vi "Read from TCP.vi"(8 "error in":errorcluster, 11 "lia host in":refnum<class "LIA Host Interface RT.lvclass">) -> (0 "error out":errorcluster, 3 "lia host out":refnum<class "LIA Host Interface RT.lvclass">)   [LabVIEW 2018, in "LIA Host Interface RT.lvclass"]
uses:
  LIA Host Interface RT.lvclass
  Properties/TcpConnection_GET.vi
  Properties/IncomingQueue_GET.vi
  Properties/LockInQueues_GET.vi
  shared/Lock-In Amplifier Example Shared.lvlib
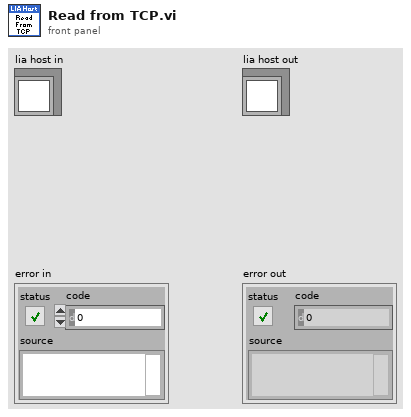
[diagram p1: front panel]
types:
  T1 = enum16{"Standard", "Buffered", "CRLF", "Immediate"}
  T2 = typedef "Lock-In Amplifier Example Shared.lvlib/message.ctl" = cluster{"command":u32, "payload":string}
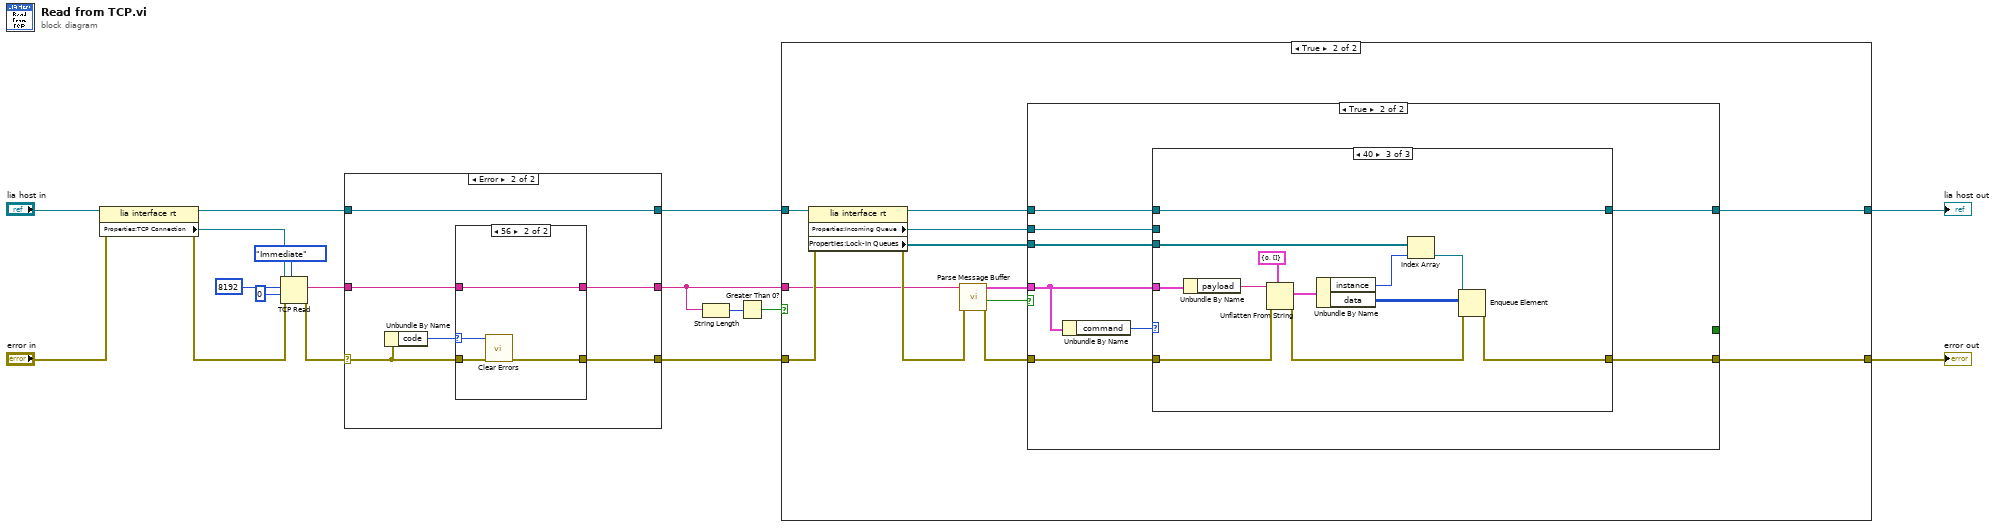
[diagram p0: block diagram]
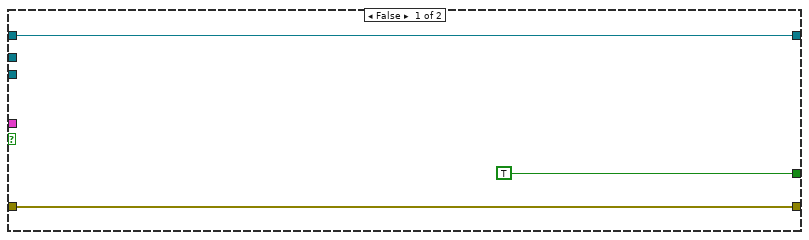
[diagram p3: hidden frame]
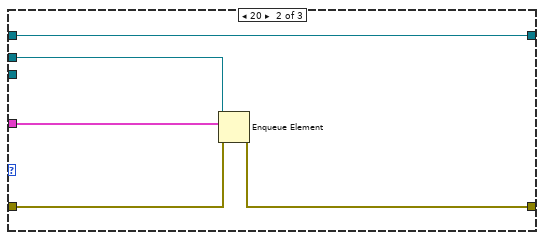
[diagram p5: hidden frame]
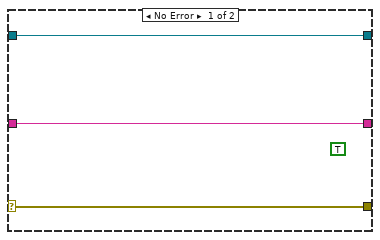
[diagram p6: hidden frame]
diagram:
  n1 = property class="lia interface rt"(reference="lia host in", error in="error in") -> (reference out=w8:refnum<class "LIA Host Interface RT.lvclass">, error out=w14:errorcluster, "Properties:TCP Connection"=w15:refnum<k5>)
  n2 = TCP Read(connection ID=w15, bytes to read=8192, error in (no error)=w14, 7:T1."Immediate" ("mode (standard)"), 9:0 ("timeout ms (25000)")) -> (data out=w5:string, error out=w7:errorcluster)  [unwired: 1 out]
  n3 = case shown="Error" w7 {
    selector: w7 -> [w19 w24]
    tunnel: [w20 w26] -> w9
    tunnel: w8 -> [w20 w26]
    tunnel: [w19 w21] -> w6
    tunnel: w5 -> [w18 w22]
    tunnel: [w18 w23] -> w4
    frame No Error {
      (unwired) TRUE
    }
    frame Error {
      n4 = Unbundle By Name(w24) -> ("code"=w25:i32)
      n5 = case shown="56" w25 {
        selector: w25 -> [_ w29]
        tunnel: w24 -> [_ w30]
        tunnel: [_ w27] -> w23
        tunnel: w22 -> [_ w27]
        tunnel: [_ w28] -> w21
        frame 0, Default {
        }
        frame 56 {
          n6 = call <vilib>:"Clear Errors.vi"("error in (no error)"=w30, "specific error code to clear (0: all)"=w29) -> ("error out"=w28:errorcluster)  [unwired: 4 in, 1 out]
        }
      }
    }
  }
  n7 = String Length(string=w4) -> (length=w1:i32)
  n8 = Greater Than 0?(x=w1) -> (x > 0?=w3:bool)
  n9 = case shown="True" w3 {
    tunnel: [w31 w44] -> w11
    tunnel: [w32 w43] -> w10
    tunnel: w9 -> [w32 w38]
    tunnel: w6 -> [w31 w37]
    tunnel: w4 -> [_ w36]
    frame False {
    }
    frame True {
      n10 = property class="lia interface rt"(reference=w38, error in=w37) -> (reference out=w42:refnum<class "LIA Host Interface RT.lvclass">, error out=w39:errorcluster, "Properties:Incoming Queue"=w41:refnum<queue>, "Properties:Lock-In Queues"=w40:refnum<queue>[])
      n11 = call "Parse Message Buffer.vi"("error in"=w39, "string in"=w36) -> ("error out"=w35:errorcluster, "valid"=w33:bool, "message"=w34:T2)  [unwired: 7 in]
      n12 = case shown="True" w33 {
        tunnel: w35 -> [w46 w50]
        tunnel: [w46 w49] -> w44
        tunnel: w34 -> [_ w48]
        tunnel: w41 -> [_ w55]
        tunnel: [w47 w54] -> w43
        tunnel: w42 -> [w47 w53]
        tunnel: w40 -> [_ w52]
        tunnel: [TRUE _] -> _
        frame False {
        }
        frame True {
          n13 = Unbundle By Name(w48) -> ("command"=w51:u32)
          n14 = case shown="40" w51 {
            tunnel: w55 -> [_ w62 _]
            tunnel: [w57 w59 w74] -> w54
            tunnel: w53 -> [w57 w59 w74]
            tunnel: w52 -> [_ _ w68]
            tunnel: w50 -> [w56 w61 w71]
            tunnel: [w56 w60 w64] -> w49
            tunnel: w48 -> [_ w58 w73]
            frame 0, Default {
            }
            frame 20 {
              n15 = Enqueue Element(queue=w62, element=w58, error in (no error)=w61) -> (error out=w60:errorcluster)  [unwired: 1 in, 2 out]
            }
            frame 40 {
              n16 = Unbundle By Name(w73) -> ("payload"=w72:string)
              n17 = Unflatten From String(type=cluster{"instance":i32, "data":i64[][]} {"instance"=0, "data"=[]}, binary string=w72, error in (no error)=w71) -> (value=w69:cluster{"instance":i32, "data":i64[][]}, error out=w65:errorcluster)  [unwired: 2 in, 1 out]
              n18 = Unbundle By Name(w69) -> ("instance"=w67:i32, "data"=w66:i64[][])
              n19 = Index Array(array=w68, index=w67) -> (element=w63:refnum<queue>)
              n20 = Enqueue Element(queue=w63, element=w66, error in (no error)=w65) -> (error out=w64:errorcluster)  [unwired: 1 in, 2 out]
            }
          }
        }
      }
    }
  }
  "error out" <- w11
  "lia host out" <- w10
